vi "Create Serial Master.vi"(4 "flow control (none)":u16(ring) items=["None", "XON/XOFF", "RTS/CTS", "XON/XOFF & RTS/CTS", "DTR/DSR", "XON/XOFF & DTR/DSR"], 5 "serial type":enum16{"RTU", "ASCII"}(ring), 6 "parity (even)":u16(ring)=2 items=["None", "Odd", "Even", "Mark", "Space"], 7 "unit ID":u8=1, 8 "error in":errorcluster, 10 "baud rate":u32=9600, 11 "VISA resource name":refnum<visa-resource-name>) -> (0 "error out":errorcluster, 3 "serial master instance":refnum<class "Modbus Master.lvclass">)   [LabVIEW 2021, in "API Main.lvlib"]
doc: "Creates a standard serial master. The transmission data unit used by the device is defined by the <B>serial type</B> input."
uses:
  API Main.lvlib
  Master/Modbus Master.lvclass
  Master Function Definition/Master Function Definition.lvclass
  Network Protocol/Network Master/Serial/Serial Master.lvclass
  D:/my_projects/projects/Algorithms/Labview/21/Modbus_v121c/Network Protocol/Network Master/Network Master.lvclass
  Transmission Data Unit/RTU/RTU Data Unit.lvclass
  D:/my_projects/projects/Algorithms/Labview/21/Modbus_v121c/Transmission Data Unit/Serial Interface/Serial Data Unit.lvclass
  Transmission Data Unit/ASCII/ASCII Data Unit.lvclass
  Transmission Data Unit/Transmission Data Unit.lvclass/Transmission Data Unit.ctl
  Transmission Data Unit/Serial Interface/Serial Data Unit.lvclass/Serial Data Unit.ctl
  Network Protocol/Network Master/Network Master.lvclass/Network Master.ctl
  Master/Modbus Master.lvclass/Modbus Master.ctl
  Transmission Data Unit/Serial Interface/Write timeout.vi
  Transmission Data Unit/Serial Interface/Write baud rate.vi
  Transmission Data Unit/Serial Interface/Write flow control.vi
  Transmission Data Unit/Serial Interface/Write parity.vi
  Transmission Data Unit/Serial Interface/Write visa resource name.vi
  Transmission Data Unit/Serial Interface/Serial Data Unit.lvclass
  D:/my_projects/projects/Algorithms/Labview/21/Modbus_v121c/Transmission Data Unit/Transmission Data Unit.lvclass
  Transmission Data Unit/Transmission Data Unit.lvclass
  Network Protocol/Network Master/Network Master.lvclass
panel:
  # "disable parity disallowed by mbspec"
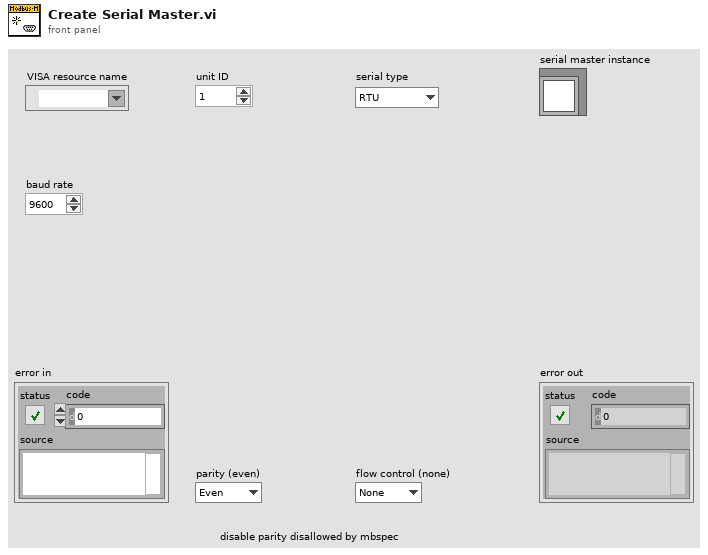
[diagram p1: front panel]
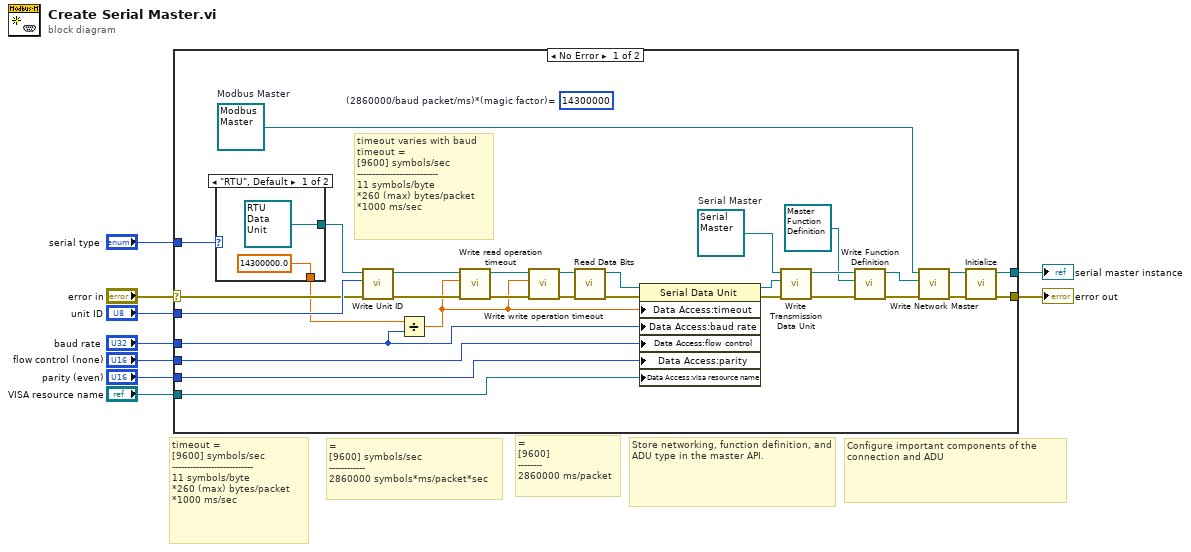
[diagram p0: block diagram]
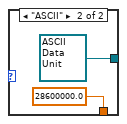
[diagram p2: hidden frame]
diagram:
  # "=\n[9600]\n--------\n2860000 ms/packet"
  # "=\n[9600] symbols/sec\n------------\n2860000 symbols*ms/packet*sec"
  # "timeout =\n[9600] symbols/sec\n---------------------------\n11 symbols/byte\n*260 (max) bytes/packet\n*1000 ms/sec"
  # "Configure important components of the connection and ADU"
  # "Store networking, function definition, and ADU type in the master API."
  n1 = case shown="No Error" "error in" {
    selector: "error in" -> [w31 w45]
    tunnel: [w40 w45] -> w8
    tunnel: [w39 _] -> w9
    tunnel: "VISA resource name" -> [w38 _]
    tunnel: "baud rate" -> [w10 _]
    tunnel: "parity (even)" -> [w37 _]
    tunnel: "flow control (none)" -> [w36 _]
    tunnel: "serial type" -> [w35 _]
    tunnel: "unit ID" -> [w33 _]
    frame No Error {
      w22 = refnum<class "Serial Master.lvclass"> refnum  # Serial Master
      (unwired) u32 14300000  # (2860000/baud packet/ms)*(magic factor)=
      w21 = refnum<class "Modbus Master.lvclass"> refnum  # Modbus Master
      # "timeout varies with baud\ntimeout =\n[9600] symbols/sec\n---------------------------\n11 symbols/byte\n*260 (max) bytes/packet\n*1000 ms/sec"
      n2 = case shown="\"RTU\", Default" w35 {
        tunnel: [refnum<class "RTU Data Unit.lvclass"> refnum ("RTU Data Unit") refnum<class "ASCII Data Unit.lvclass"> refnum ("ASCII Data Unit")] -> w34
        tunnel: [14300000.0 ("x") 28600000.0 ("x")] -> w27
        frame "RTU", Default {
        }
        frame "ASCII" {
        }
      }
      n3 = call "Write Unit ID.vi"("error in"=w31, "unit ID"=w33, "transmission data unit in"=w34) -> ("error out"=w28:errorcluster, "transmission data unit out"=w32:refnum<class "Serial Data Unit.lvclass">)  [unwired: 7 in]
      n4 = Divide(x=w27, y=w10) -> (x/y=w24:dbl)
      n5 = call "Write read operation timeout.vi"("error in (no error)"=w28, "read operation timeout"=w24, "transmission data unit in"=w32) -> ("error out"=w29:errorcluster, "transmission data unit out"=w30:refnum<class "Serial Data Unit.lvclass">)  [unwired: 7 in]
      n6 = call "Write write operation timeout.vi"("error in (no error)"=w29, "write operation timeout"=w24, "transmission data unit in"=w30) -> ("error out"=w26:errorcluster, "transmission data unit out"=w25:refnum<class "Serial Data Unit.lvclass">)  [unwired: 7 in]
      n7 = call-dynamic "Read Data Bits.vi"("error in (no error)"=w26, "Serial Data Unit in"=w25) -> ("error out"=w23:errorcluster, "Serial Data Unit out"=w13:refnum<class "Serial Data Unit.lvclass">)  [unwired: 7 in, 1 out]
      n8 = property class="Serial Data Unit"(reference=w13, error in=w23, "Data Access:timeout"=w24, "Data Access:baud rate"=w10, "Data Access:flow control"=w36, "Data Access:parity"=w37, "Data Access:visa resource name"=w38) -> (reference out=w11:refnum<class "Serial Data Unit.lvclass">, error out=w12:errorcluster)
      n9 = call "Write Transmission Data Unit.vi"("error in (no error)"=w12, "Transmission Data Unit"=w11, "Network Master in"=w22) -> ("error out"=w16:errorcluster, "Network Master out"=w18:refnum<class "Serial Master.lvclass">)  [unwired: 7 in]
      n10 = call "Write Function Definition.vi"("error in"=w16, "master function definition"=refnum<class "Master Function Definition.lvclass"> refnum ("Master Function Definition"), "Modbus master in"=w18) -> ("error out"=w15:errorcluster, "Modbus master out"=w17:refnum<class "Serial Master.lvclass">)  [unwired: 7 in]
      n11 = call "Write Network Master.vi"("error in"=w15, "Network Master"=w17, "Modbus master in"=w21) -> ("error out"=w19:errorcluster, "Modbus master out"=w20:refnum<class "Modbus Master.lvclass">)  [unwired: 7 in]
      n12 = call-dynamic "Initialize.vi"("error in (no error)"=w19, "Modbus master in"=w20) -> ("error out"=w40:errorcluster, "Modbus master out"=w39:refnum<class "Modbus Master.lvclass">)  [unwired: 8 in]
    }
    frame Error {
    }
  }
  "error out" <- w8
  "serial master instance" <- w9
